vi "MotorTrifasico.vi"() -> ()   [LabVIEW 2010]
uses:
  <vilib>/Platform/TimedLoop/XDataNode/XDataNode.xnode
  <vilib>/Platform/TimedLoop/XDataNode/timing_clust.ctl
  <vilib>/Platform/TimedLoop/XDataNode/nitl_modes.ctl
  <vilib>/Platform/TimedLoop/XDataNode/wakeup.ctl
  <vilib>/Instr/_visa.llb/VISA Configure Serial Port (Instr).vi
  <vilib>/addons/System Identification/Parametric Estimation.llb/SI Estimate State-Space Model (SISO Array).vi
  <vilib>/addons/System Identification/Model Conversion.llb/SI Convert to Zero-Pole-Gain Model of CDT.vi
  <vilib>/addons/Control Design/_Utility/Model Viewer.llb/Model Viewer SubVI/cd_Draw Zero-Pole-Gain Equation (ZPK).vi
  <vilib>/addons/System Identification/Model Analysis.llb/SI Model Simulation (SISO Array).vi
  <vilib>/Platform/TimedLoop/XDataNode/XDNodeRunTimeDep.lvlib
  <vilib>/addons/System Identification/NI_SysID.lvlib
  <vilib>/addons/Control Design/_Utility/NI_CD_Model Viewer.lvlib
panel:
  out "error out":errorcluster
  in  "stop":bool
  in  "Tab Control":T1(tab)
  out "Manual":bool
  out "FRECUENCIA":dbl(knob) scale=0.0..30.0
  out "Vueltas/600ms 2":dbl(knob) scale=0.0..20.0
  out "1 2":bool
  out "2 2":bool
  out "3 2":bool
  out "4 2":bool
  out "RPM 2":dbl(graph)
  in  "Period                :":i64=1000
  in  "Flow control    :":u16(ring) items=["None"=0, "XON/XOFF"=1, "RTS/CTS"=2, "DTR/DSR"=4]
  in  "Stop bits         :":u16(ring)=10 items=["1.0"=10, "1.5"=15, "2.0"=20]
  in  "Paridad            :":u16(ring) items=["None", "Odd", "Even", "Mark", "Space"]
  in  "Data bits          :":u16=8 min=5 max=8 step=1
  in  "VISA resource : name:":refnum<visa-resource-name>="COM1"
  in  "Baud rate         :":u32=9600
  out "Read buffer":string
  in  "control":dbl(slide) scale=0.0..30.0
  out "ind":dbl
  out "Ajuste 2":dbl(slide) scale=0.0..30.0
  out "RPM":dynamicdata(graph)
  in  "Automatico":bool
  in  "Ajuste":dbl(slide) scale=0.0..1.0
  in  "SET RPM":dbl(knob) scale=0.0..800.0
  out "4":bool
  out "3":bool
  out "2":bool
  out "1":bool
  out "HZ":dbl(knob) scale=0.0..30.0
  out "Vueltas/600ms":dbl(knob) scale=0.0..20.0
  out "Waveform Graph":dbl[][](graph)=[[-2.67, 1853.997, 2087.33, 2090.663, 2090.663, 2097.33, 2093.997, 2093.997, 2093.997, 2097.33, 2093.997, 857.33, 97.33, 83.997, 90.663, 93.997, 83.997, 87.33, 93.997, 90.663], [-166.61063012940264, 1790.7492530367795, 1987.1989621593734, 1957.2279393678514, 1939.890791703056, 1938.4615637891961, 1930.134134639174, 1927.776406485906, 1926.5639511296883, 1929.683064580092, 1931.5209671870887, 687.235820612786, -91.92682182294811, -68.72120107004889, -41.603445425021405, -27.76373407264424, -33.80087603938517, -27.38837763115518, -18.529043853060102, -21.566730744936933]]
  out "MODELO MATEMÁTICO PLANTA - SS":picture
  in  "nùmero de estados":i32=1
  out "estimulo":dbl[](array[numeric])
  out "respuesta":dbl[](array[numeric])
  out "ind":dbl
  out "String":string
  in  "i":dbl
  out "Numeric":dbl
  # "Motor Trifasico 480Vac"
  # "Configuracion Serial"
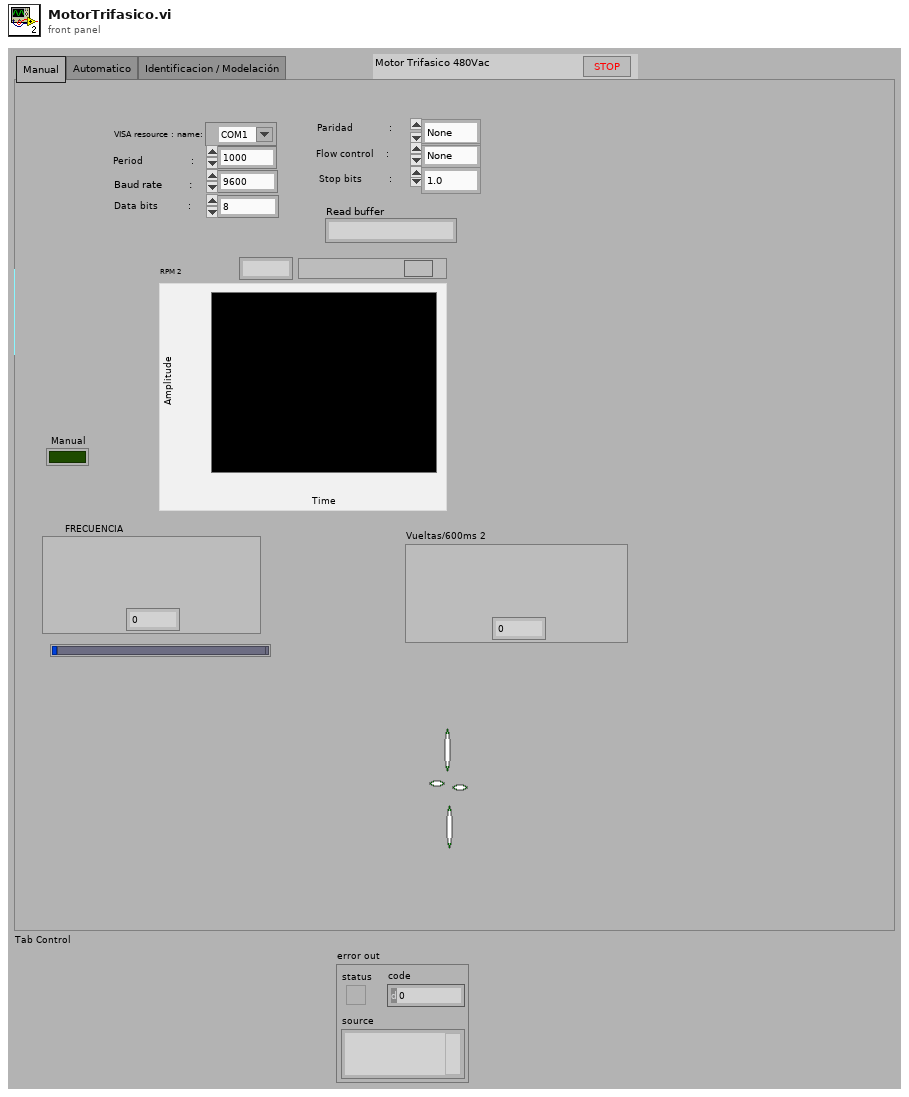
[diagram p1: front panel]
types:
  T1 = enum32{"Manual", "Automatico", "Identificacion / Modelación"}
  T2 = typedef "XDNodeRunTimeDep.lvlib/timing_clust.ctl" = cluster{"Expected End [f-1]":u64, "Actual End [f-1]":u64, "Finished Late? [f-1]":bool, "Expected End [i-1]":u64, "Actual End [i-1]":u64, "Finished Late? [i-1]":bool, "Expected Start [i]":u64, "Actual Start [i]":u64, "Expected Start [f]":u64, "Actual Start [f]":u64, "Source Name":string, "Structure Name":string, "Period":i64, "Deadline":i64, "Offset":i64, "Start":i64, "Priority":i32, "Timeout":i32, "Mode":T3, "Wakeup Reason":T4, "Error":errorcluster, "Source Type":string, "Secondary Source Type":string, "Global End Time":u64, "Global Start Time":u64, "Frame Duration":u64, "Iteration Duration":u64, "Assigned CPU":i32, "I/O Scan Engine Mode":u32}
  T3 = typedef "XDNodeRunTimeDep.lvlib/nitl_modes.ctl" = enum32{"No Change", "Process missed periods, maintain original phase", "Discard missed periods, maintain original phase", "Process missed periods, ignore original phase", "Discard missed periods, ignore original phase"}
  T4 = typedef "XDNodeRunTimeDep.lvlib/wakeup.ctl" = enum32{"Normal", "Aborted", "Asynchronous wakeup", "Timing source error", "Timed loop error", "Timeout"}
  T5 = typedef "NI_SysID.lvlib/si_generic model.ctl" = cluster{"attributes":cluster{"version":string, "model type":T6, "input names":string[], "output names":string[], "notes":string}, "coefficients":cluster{"A ":dbl[][][], "B":dbl[][][], "F":dbl[][][], "C":dbl[][][], "D":dbl[][][]}, "std deviations":cluster{"A ":dbl[][][], "B":dbl[][][], "F":dbl[][][], "C":dbl[][][], "D":dbl[][][]}, "coefficients covariance":dbl[][][], "noise variance":dbl[][], "fs":dbl, "system info":cluster{"number of inputs":i32, "number of outputs":i32, "A order":i32[][], "B order":i32[][], "F order":i32[][], "C order":i32[][], "D order":i32[][], "Delays":i32[][]}, "kalman gain":dbl[][], "initial state":dbl[], "trans func":cluster{"betas":dbl[], "alphas":dbl[]}[][], "zeros-poles":cluster{"zeros":cdb[], "poles":cdb[], "gain":dbl}[][], "std of trans func":cluster{"betas":dbl[], "alphas":dbl[]}[][], "std of zeros-poles":cluster{"zeros":cdb[], "poles":cdb[], "gain":dbl}[][], "trans func (noise)":cluster{"betas":dbl[], "alphas":dbl[]}[][], "std of trans func (noise)":cluster{"betas":dbl[], "alphas":dbl[]}[][], "zeros-poles (noise)":cluster{"zeros":cdb[], "poles":cdb[], "gain":dbl}[][], "std of zeros-poles (noise)":cluster{"zeros":cdb[], "poles":cdb[], "gain":dbl}[][], "Symbolic State Space Model":cluster{"Symbolic A":string[][], "Symbolic B":string[][], "Symbolic C":string[][], "Symbolic D":string[][], "Symbolic K":string[][], "Symbolic Initial State":string[]}, "delay":dbl[][], "variables":T7, "grey trans func spec":cluster{"orders of TF model":cluster{" num order":i32, "den order":i32}, "# of zeros/poles at origin":cluster{"zeros/poles":u16, "number ":i32}, "delay initial?":bool, "gain initial?":bool}}
  T6 = typedef "NI_SysID.lvlib/SI Model Type.ctl" = u16
  T7 = typedef "NI_SysID.lvlib/si_variables.ctl" = cluster{"name":string, "initial guess":dbl, "upper limit":dbl, "lower limit":dbl, "value":dbl}[]
  T8 = typedef "NI_LinSys_Model Typedefs.lvlib/CD Zero-Pole-Gain Model (MIMO).ctl" = cluster{"properties":T9, "zero-pole-gain(s)":T10[][]}
  T9 = typedef "NI_LinSys_Model Typedefs.lvlib/CD General Elements.ctl" = cluster{"Model name":string, "Input names":string[], "Output names":string[], "Input Delays":dbl[], "Output Delays":dbl[], "Sampling Time":dbl, "Notes":string}
  T10 = typedef "NI_LinSys_Model Typedefs.lvlib/CD Zero-Pole-Gain Model (SISO).ctl" = cluster{"Gain":dbl, "Zeros":cdb[], "Poles":cdb[], "delay":dbl}
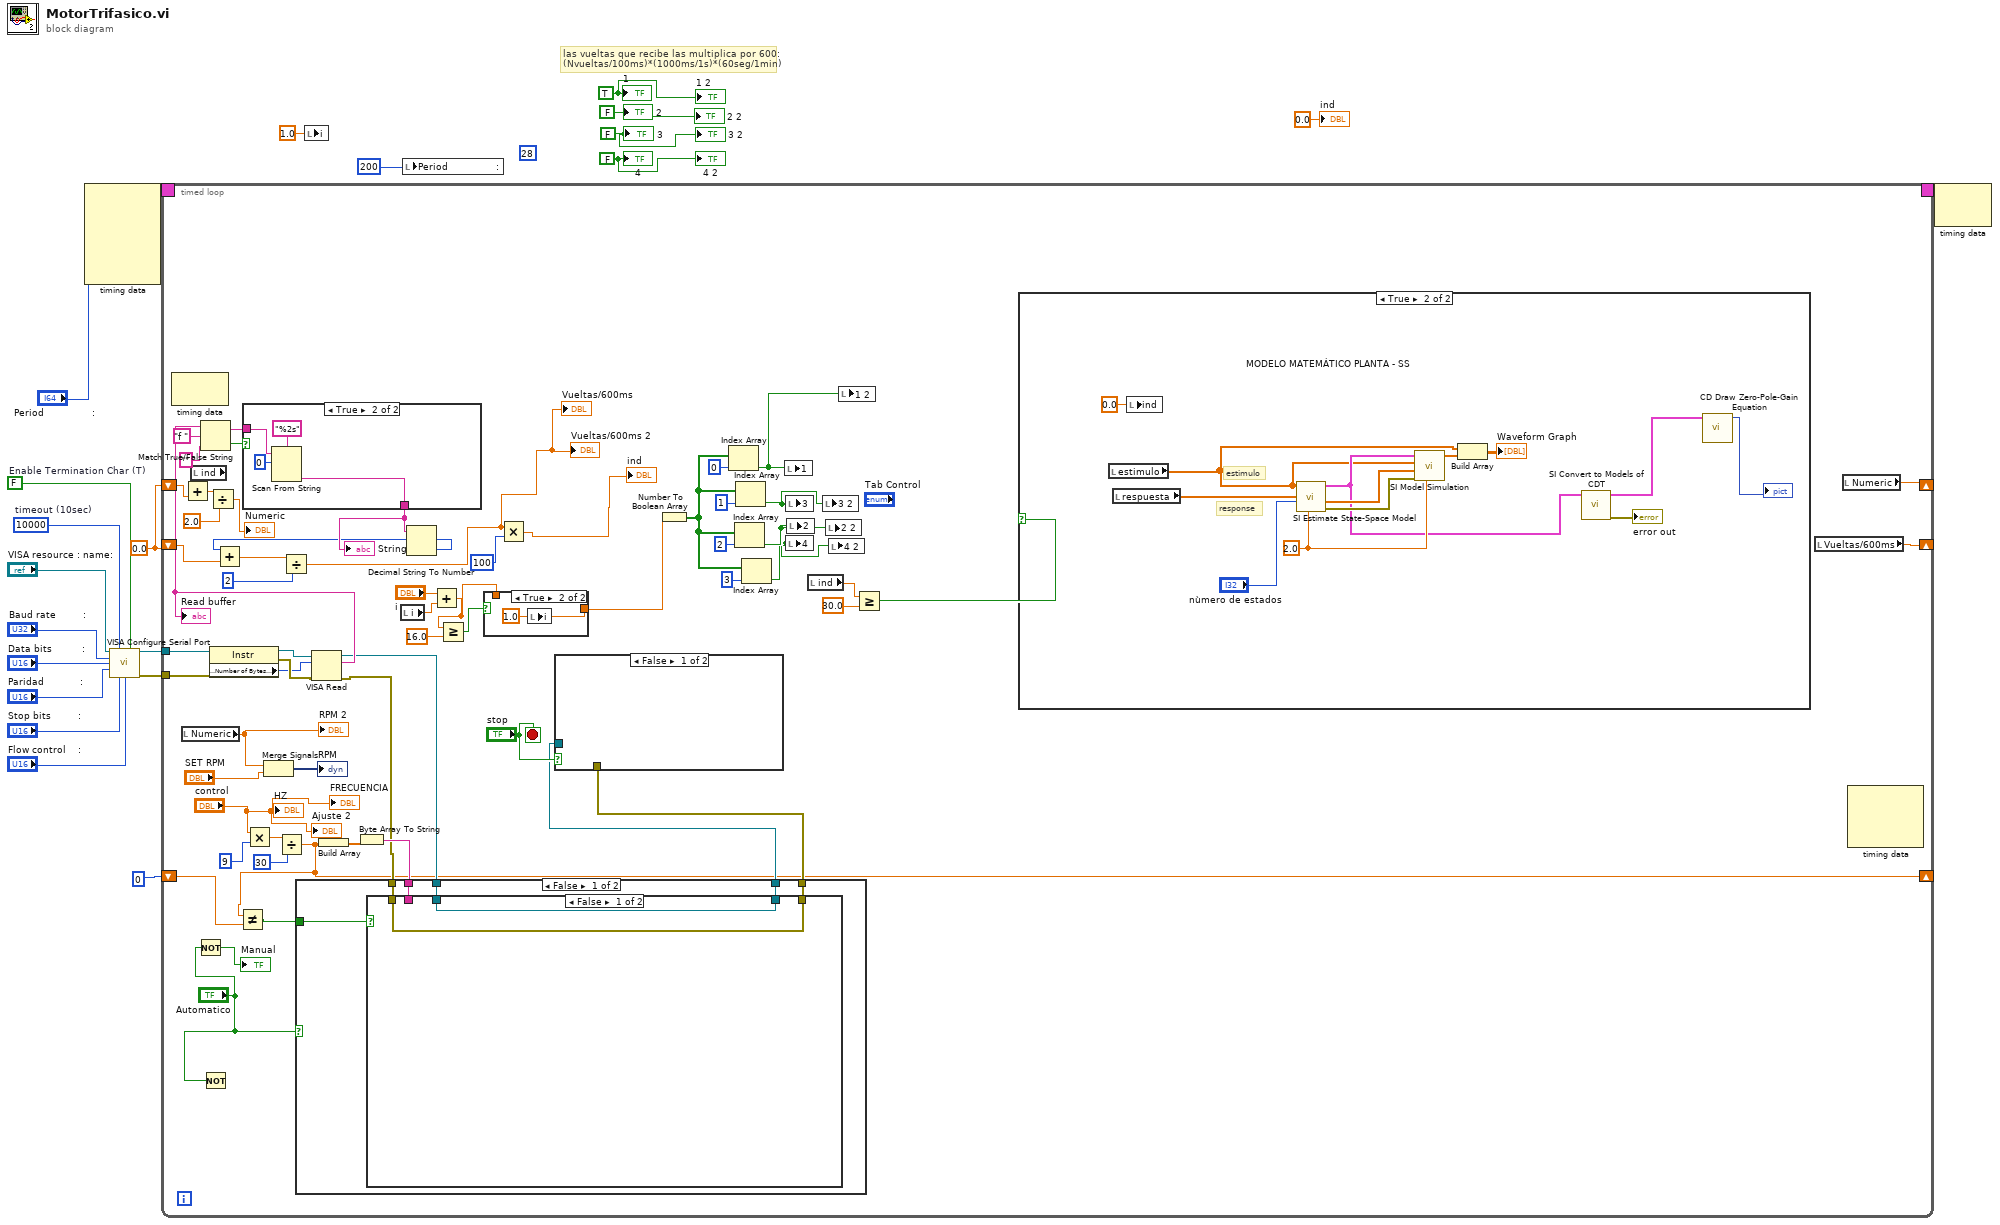
[diagram p0: block diagram]
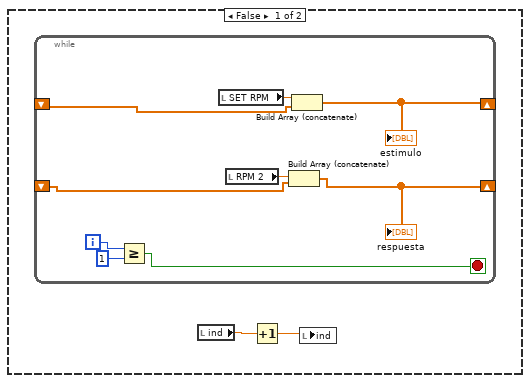
[diagram p2: hidden frame]
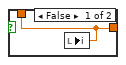
[diagram p3: hidden frame]
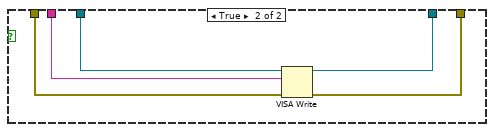
[diagram p4: hidden frame]
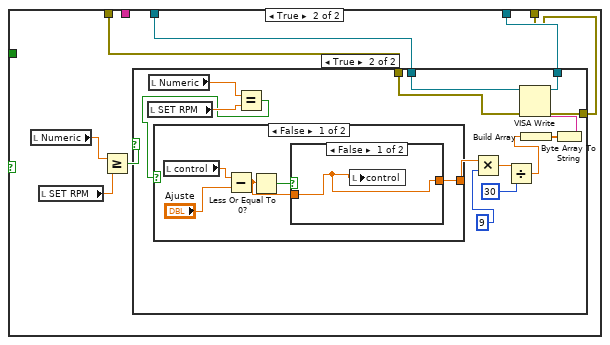
[diagram p5: hidden frame]
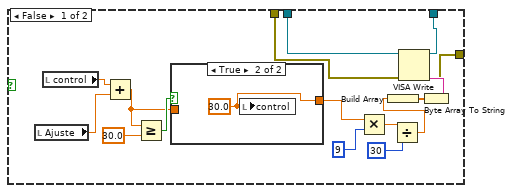
[diagram p6: hidden frame]
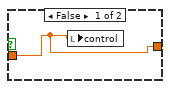
[diagram p7: hidden frame]
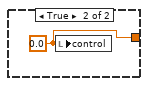
[diagram p8: hidden frame]
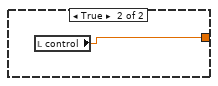
[diagram p9: hidden frame]
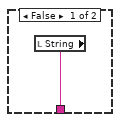
[diagram p10: hidden frame]
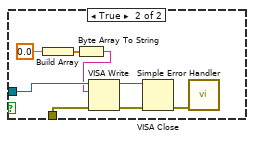
[diagram p11: hidden frame]
diagram:
  w6 = 0.0 ("Vueltas/600ms")
  w2 = FALSE ("4")
  w3 = FALSE ("3")
  w4 = FALSE ("2")
  w5 = TRUE ("1")
  (unwired) u8 28 ("Set- Point\n Temperatura Exterior (C)")
  w16 = FALSE  # Enable Termination Char (T)
  w17 = u32 10000  # timeout (10sec)
  # "las vueltas que recibe las multiplica por 600:\n(Nvueltas/100ms)*(1000ms/1s)*(60seg/1min)"
  n1 = node-c288("Period                :") -> (w22:T2)  [unwired: 4 in]
  n2 = call-poly "VISA Configure Serial Port"("VISA resource name"="VISA resource : name:", "timeout (10sec)"=w17, "Enable Termination\nChar (T)"=w16, "baud rate (9600)"="Baud rate         :", "data bits (8)"="Data bits          :", "parity (0:none)"="Paridad            :", "stop bits (10: 1 bit)"="Stop bits         :", "flow control (0:none)"="Flow control    :") -> ("VISA resource name out"=w12:refnum<visa-resource-name>, "error out"=w11:errorcluster)  [unwired: 6 in]
  n3 = timed-loop {
    timing: w22 -> [_]
    timing-out: [_] -> w21
    tunnel: w12 -> [w77]
    tunnel: w11 -> [w76]
    shift-right: [w65] -> _
    shift-left: u8 0 ("Set- Point\n Temperatura Exterior (C)") -> [w64]
    shift-right: [w41] -> _
    shift-left: w6 -> [w45]
    shift-right: [w36] -> _
    shift-left: w6 -> [w40]
    stop <- "stop" stop-if-true
    n4 = node-c288() -> ()  [unwired: 1 in, 1 out]
    n5 = local read "Numeric"() -> (w34:dbl)
    "RPM 2" <- w34
    n6 = local read "ind"() -> (w37:dbl)
    n7 = Add(x=w37, y=w40) -> (x+y=w39:dbl)
    n8 = Not(x="Automatico") -> (.not. x?=→"Manual":bool)
    n9 = Not(x="Automatico") -> ()  [unwired: 1 out]
    n10 = Divide(x=w39, y=2.0) -> (x/y=→"Numeric":dbl)
    n11 = property class="Instr"(reference=w77, error in=w76) -> (reference out=w78:refnum<visa-resource-name>, error out=w84:errorcluster, "Serial Settings:Number of Bytes at Serial Port"=w83:u32)
    n12 = Multiply(x="control", y=u8 9) -> (x*y=w69:dbl)
    n13 = Merge Signals(w34, "SET RPM") -> (→"RPM":dynamicdata)
    n14 = Divide(x=w69, y=u8 30) -> (x/y=w65:dbl)
    n15 = Not Equal?(x=w65, y=w64) -> (x != y?=w66:bool)
    n16 = VISA Read(VISA resource name=w78, byte count=w83, error in (no error)=w84) -> (VISA resource name out=w74:refnum<visa-resource-name>, read buffer=w81:string, error out=w72:errorcluster)  [unwired: 1 out]
    "Read buffer" <- w81
    n17 = Match True/False String(2:"" ("false string"), 3:"f " ("true string"), 4:w81) -> (0:w49:bool, 1:w50:string)
    n18 = case shown="True" w49 {
      tunnel: [w171 w172] -> w48
      tunnel: w50 -> [_ w173]
      frame False {
        n19 = local read "String"() -> (w171:string)
      }
      frame True {
        n20 = Scan From String(format string="%2s", input string=w173, initial scan location=u32 0) -> (output 1=w172:string)  [unwired: 2 in, 3 out]
      }
    }
    "String" <- w48
    n21 = Build Array(w65) -> (w75:dbl[])
    n22 = Byte Array To String(unsigned byte array=w75) -> (string=w73:string)
    n23 = case shown="False" "Automatico" {
      tunnel: w74 -> [w116 w128]
      tunnel: w73 -> [w115 _]
      tunnel: w72 -> [w114 w127]
      tunnel: [w113 w125] -> w71
      tunnel: [w112 w126] -> w67
      tunnel: w66 -> [w111 _]
      frame False {
        n24 = case shown="False" w111 {
          tunnel: w116 -> [w118 w123]
          tunnel: w115 -> [_ w122]
          tunnel: w114 -> [w117 w121]
          tunnel: [w118 w120] -> w112
          tunnel: [w117 w119] -> w113
          frame False {
          }
          frame True {
            n25 = VISA Write(VISA resource name=w123, write buffer=w122, error in (no error)=w121) -> (VISA resource name out=w120:refnum<visa-resource-name>, error out=w119:errorcluster)  [unwired: 1 out]
          }
        }
      }
      frame True {
        n26 = local read "Numeric"() -> (w124:dbl)
        n27 = local read "SET RPM"() -> (w129:dbl)
        n28 = Greater Or Equal?(x=w124, y=w129) -> (x >= y?=w130:bool)
        n29 = case shown="True" w130 {
          tunnel: w128 -> [w142 w160]
          tunnel: w127 -> [w141 w159]
          tunnel: [w140 w158] -> w126
          tunnel: [w139 w157] -> w125
          frame False {
            n30 = local read "Ajuste"() -> (w143:dbl)
            n31 = local read "control"() -> (w146:dbl)
            n32 = Add(x=w146, y=w143) -> (x+y=w137:dbl)
            n33 = Greater Or Equal?(x=w137, y=30.0) -> (x >= y?=w138:bool)
            n34 = case shown="True" w138 {
              tunnel: w137 -> [w147 _]
              tunnel: [w147 w148] -> w132
              frame False {
                n35 = local write "control"(w147) -> ()
              }
              frame True {
                w148 = 30.0 ("control")
                n36 = local write "control"(w148) -> ()
              }
            }
            n37 = Multiply(x=w132, y=u8 9) -> (x*y=w134:dbl)
            n38 = Divide(x=w134, y=u8 30) -> (x/y=w131:dbl)
            n39 = Build Array(w131) -> (w144:dbl[])
            n40 = Byte Array To String(unsigned byte array=w144) -> (string=w145:string)
            n41 = VISA Write(VISA resource name=w142, write buffer=w145, error in (no error)=w141) -> (VISA resource name out=w140:refnum<visa-resource-name>, error out=w139:errorcluster)  [unwired: 1 out]
          }
          frame True {
            n42 = local read "SET RPM"() -> (w151:dbl)
            n43 = local read "Numeric"() -> (w152:dbl)
            n44 = Equal?(x=w152, y=w151) -> (x = y?=w149:bool)
            n45 = case shown="False" w149 {
              tunnel: [w163 w170] -> w154
              frame False {
                n46 = local read "control"() -> (w167:dbl)
                n47 = Subtract(x=w167, y="Ajuste") -> (x-y=w164:dbl)
                n48 = Less Or Equal To 0?(x=w164) -> (x <= 0?=w165:bool)
                n49 = case shown="False" w165 {
                  tunnel: w164 -> [w168 _]
                  tunnel: [w168 w169] -> w163
                  frame False {
                    n50 = local write "control"(w168) -> ()
                  }
                  frame True {
                    w169 = 0.0 ("control")
                    n51 = local write "control"(w169) -> ()
                  }
                }
              }
              frame True {
                n52 = local read "control"() -> (w170:dbl)
              }
            }
            n53 = Multiply(x=w154, y=u8 9) -> (x*y=w156:dbl)
            n54 = Divide(x=w156, y=u8 30) -> (x/y=w153:dbl)
            n55 = Build Array(w153) -> (w161:dbl[])
            n56 = Byte Array To String(unsigned byte array=w161) -> (string=w162:string)
            n57 = VISA Write(VISA resource name=w160, write buffer=w162, error in (no error)=w159) -> (VISA resource name out=w158:refnum<visa-resource-name>, error out=w157:errorcluster)  [unwired: 1 out]
          }
        }
      }
    }
    n58 = local read "i"() -> (w55:dbl)
    n59 = Decimal String To Number(string=w48) -> (number=w46:i32)  [unwired: 2 in, 1 out]
    n60 = Add(x=w46, y=w45) -> (x+y=w44:dbl)
    n61 = Divide(x=w44, y=2) -> (x/y=w23:dbl)
    "Vueltas/600ms" <- w23
    "Vueltas/600ms 2" <- w23
    n62 = Add(x="i", y=w55) -> (x+y=w51:dbl)
    n63 = Greater Or Equal?(x=w51, y=16.0) -> (x >= y?=w54:bool)
    n64 = case shown="True" w54 {
      tunnel: [w109 w110] -> w52
      tunnel: w51 -> [w109 _]
      frame False {
        n65 = local write "i"(w109) -> ()
      }
      frame True {
        w110 = 1.0 ("i")
        n66 = local write "i"(w110) -> ()
      }
    }
    n67 = Multiply(x=w23, y=100) -> (x*y=→"ind":dbl)
    n68 = case shown="False" "stop" {
      tunnel: w67 -> [_ w180]
      tunnel: w71 -> [_ w179]
      frame False {
      }
      frame True {
        n69 = Build Array(0.0 ("element")) -> (w178:dbl[])
        n70 = Byte Array To String(unsigned byte array=w178) -> (string=w176:string)
        n71 = VISA Write(VISA resource name=w180, write buffer=w176, error in (no error)=w179) -> (VISA resource name out=w182:refnum<visa-resource-name>, error out=w181:errorcluster)  [unwired: 1 out]
        n72 = VISA Close(VISA resource name=w182, error in (no error)=w181) -> (error out=w183:errorcluster)
        n73 = call <vilib>:"Simple Error Handler.vi"("error in (no error)"=w183) -> ()  [unwired: 4 in, 5 out]
      }
    }
    n74 = Number To Boolean Array(number=w52) -> (Boolean array=w57:bool[])
    n75 = Index Array(array=w57, index=0) -> (element=w33:bool)
    n76 = Index Array(array=w57, index=2) -> (element=w31:bool)
    n77 = Index Array(array=w57, index=1) -> (element=w32:bool)
    n78 = Index Array(array=w57, index=3) -> (element=w30:bool)
    n79 = local write "1"(w33) -> ()
    n80 = local write "3"(w32) -> ()
    n81 = local write "4"(w30) -> ()
    n82 = local write "2"(w31) -> ()
    n83 = local read "ind"() -> (w25:dbl)
    n84 = local write "3 2"(w32) -> ()
    n85 = local write "2 2"(w31) -> ()
    n86 = local write "4 2"(w30) -> ()
    n87 = local write "1 2"(w33) -> ()
    n88 = Greater Or Equal?(x=w25, y=30.0) -> (x >= y?=w26:bool)
    n89 = case shown="True" w26 {
      frame False {
        n90 = while {
          shift-right: [w92] -> _
          shift-left: _ -> [w91]
          shift-right: [w93] -> _
          shift-left: _ -> [w90]
          i -> [w89]
          stop <- w88 stop-if-true
          n91 = Greater Or Equal?(x=w89, y=1) -> (x >= y?=w88:bool)
          n92 = local read "SET RPM"() -> (w95:dbl)
          n93 = local read "RPM 2"() -> (w94:dbl)
          n94 = Build Array (concatenate)(w94, w90) -> (w93:dbl[])
          "respuesta" <- w93
          n95 = Build Array (concatenate)(w95, w91) -> (w92:dbl[])
          "estimulo" <- w92
        }
        n96 = local read "ind"() -> (w85:dbl)
        n97 = Increment(x=w85) -> (x+1=w86:dbl)
        n98 = local write "ind"(w86) -> ()
      }
      frame True {
        w106 = 2.0 ("sampling rate")
        # "response"
        # "estimulo"
        n99 = local read "estimulo"() -> (w98:dbl[])
        n100 = local read "respuesta"() -> (w99:dbl[])
        n101 = local write "ind"(0.0 ("ind")) -> ()
        n102 = call-poly <vilib>:"SI Estimate State-Space Model.vi"("sampling rate"=w106, "number of states"="nùmero de estados", "response signal"=w99, "stimulus signal"=w98) -> ("error out"=w105:errorcluster, "noise"=w104:dbl[], "system model out"=w100:T5)  [unwired: 2 in, 3 out]
        n103 = call-poly <vilib>:"SI Model Simulation.vi"("sampling rate"=w106, "error in (no error)"=w105, "noise"=w104, "stimulus signal"=w98, "system model"=w100) -> ("response"=w102:dbl[])  [unwired: 6 out]
        n104 = Build Array(w98, w102) -> (→"Waveform Graph":dbl[][])
        n105 = call-poly <vilib>:"SI Convert to Models of CDT.vi"("system model"=w100) -> ("error out"=→"error out":errorcluster, "zero-pole-gain model"=w97:T8)  [unwired: 2 in, 7 out]
        n106 = call-poly <vilib>:"CD Draw Zero-Pole-Gain Equation.vi"("Zero-Pole-Gain Model"=w97) -> ("Equation"=→"MODELO MATEMÁTICO PLANTA - SS":picture)  [unwired: 8 in, 2 out]
      }
    }
    n107 = local read "Vueltas/600ms"() -> (w41:dbl)
    n108 = local read "Numeric"() -> (w36:dbl)
    n109 = node-c288() -> ()  [unwired: 3 in, 1 out]
    "HZ" <- "control"
    "FRECUENCIA" <- "control"
    "Ajuste 2" <- "control"
  }
  n110 = local write "i"(1.0 ("i")) -> ()
  n111 = local write "Period                :"(i64 200 ("Period")) -> ()
  n112 = node-c288(w21) -> ()  [unwired: 1 out]
  "1" <- w5
  "2" <- w4
  "3" <- w3
  "4" <- w2
  "1 2" <- w5
  "4 2" <- w2
  "3 2" <- w3
  "2 2" <- w4
  "ind" <- 0.0 ("ind")
